vi "Mindsensors SumoEyes Config.vi"(10 "Node Data":T2) -> ()   [LabVIEW 2010]
uses:
  Datatypes/Node.ctl
  UI Controls/PlugInControls/Pluginbackground.ctl
  <vilib>/NXT/Subs/LVHSConnector.ctl
  <vilib>/Utility/miscctls.llb/LVPointTypeDef.ctl
  <vilib>/NXT/Block Support/HWPage.SensorMode.ctl
  <vilib>/NXT/Block Support/HWPage.SensorType.ctl
  ConvertNodeAddrSensor.vi
  SavePendingGlobal.vi
panel:
  in  "Ring":u16(ring)=5 items=["short"=5, "long"=6]
  out "?":ext format="%#.2g"
  in  "NXT Port":string
  out "Both 2":bool
  out "Right 2":bool
  out "Left 2":bool
  out "Both":bool
  out "Right":bool
  out "Left":bool
  in  "Range":string
  out "Reading":i16=45
  in  "NXT":T1
  in  "Name":string
  out "Headline":string="Type (auto populated)"
  in  "Sensor Parameters":string
  in  "Reset":bool
  in  "Save":bool
  in  "Stop":bool
  out "Background":T3=TRUE
  # "<- No controls below this line"
  # "Common controls such as Buttons, Rings, Sliders, Graphs, Decorations, etc can be found in the <labview>\\Targets\\NI\\NXT\\NXT Toolkit\\Schematic Editor\\UI Controls\\Plugin Controls\\ folder. Use these controls when possible to ensure a consistent look and feel with LabVIEW Education Edition."
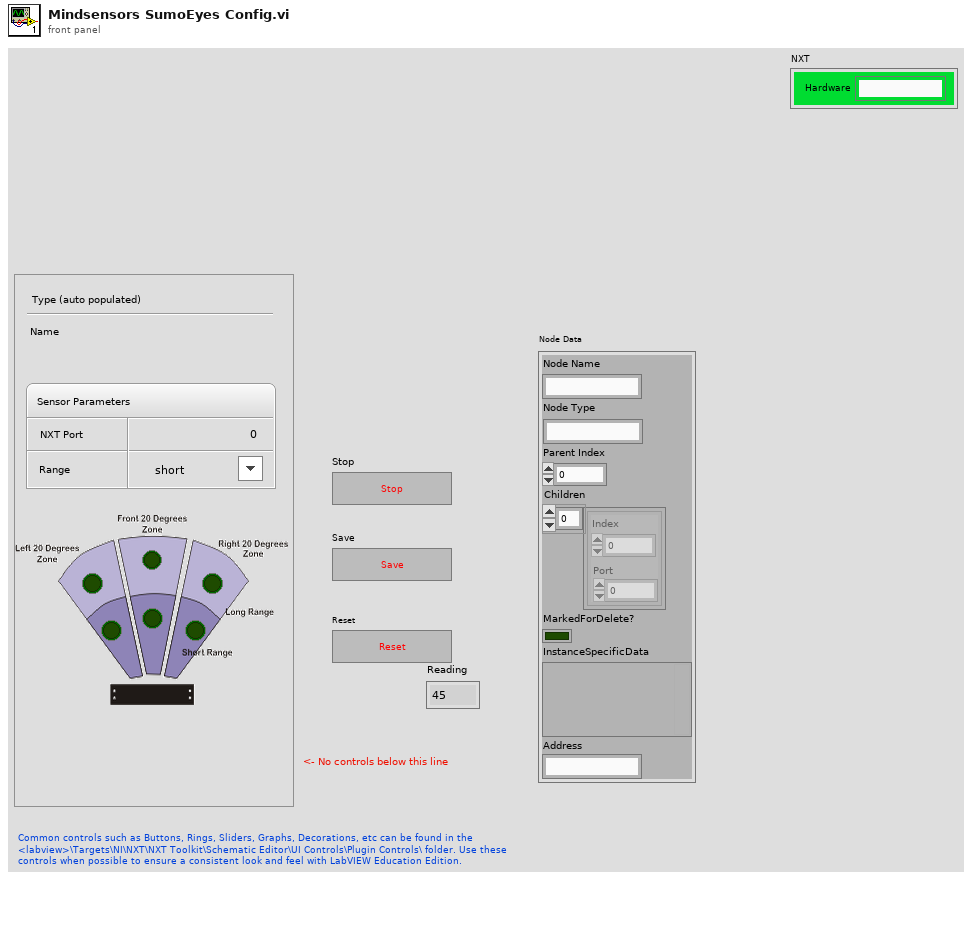
[diagram p1: front panel]
types:
  T1 = typedef "LVHSConnector.ctl" = cluster{"Hardware":string, "Flattened String":string}
  T2 = typedef "Node.ctl" = cluster{"Node Name":string, "Node Type":string, "Parent Index":i16, "Children":cluster{"Index":u16, "Port":u16}[], "MarkedForDelete?":bool, "InstanceSpecificData":variant, "Address":string}
  T3 = typedef "Pluginbackground.ctl" = bool
  T4 = typedef "LVPointTypeDef.ctl" = cluster{"Horizontal":i16, "Vertical":i16}
  T5 = enum8{"Enabled", "Disabled", "Disabled and Grayed Out"}
  T6 = typedef "HWPage.SensorMode.ctl" = u8
  T7 = typedef "HWPage.SensorType.ctl" = u8
  T8 = typedef "NXT_InputPort.ctl" = u8
  T9 = typedef "nxt.ctl" = cluster{"nxtHandle":u32, "fileHandle":u32, "fileIterHandle":u32, "moduleHandle":u32, "modIterHandle":u32, "nxtIterHandle":u32}
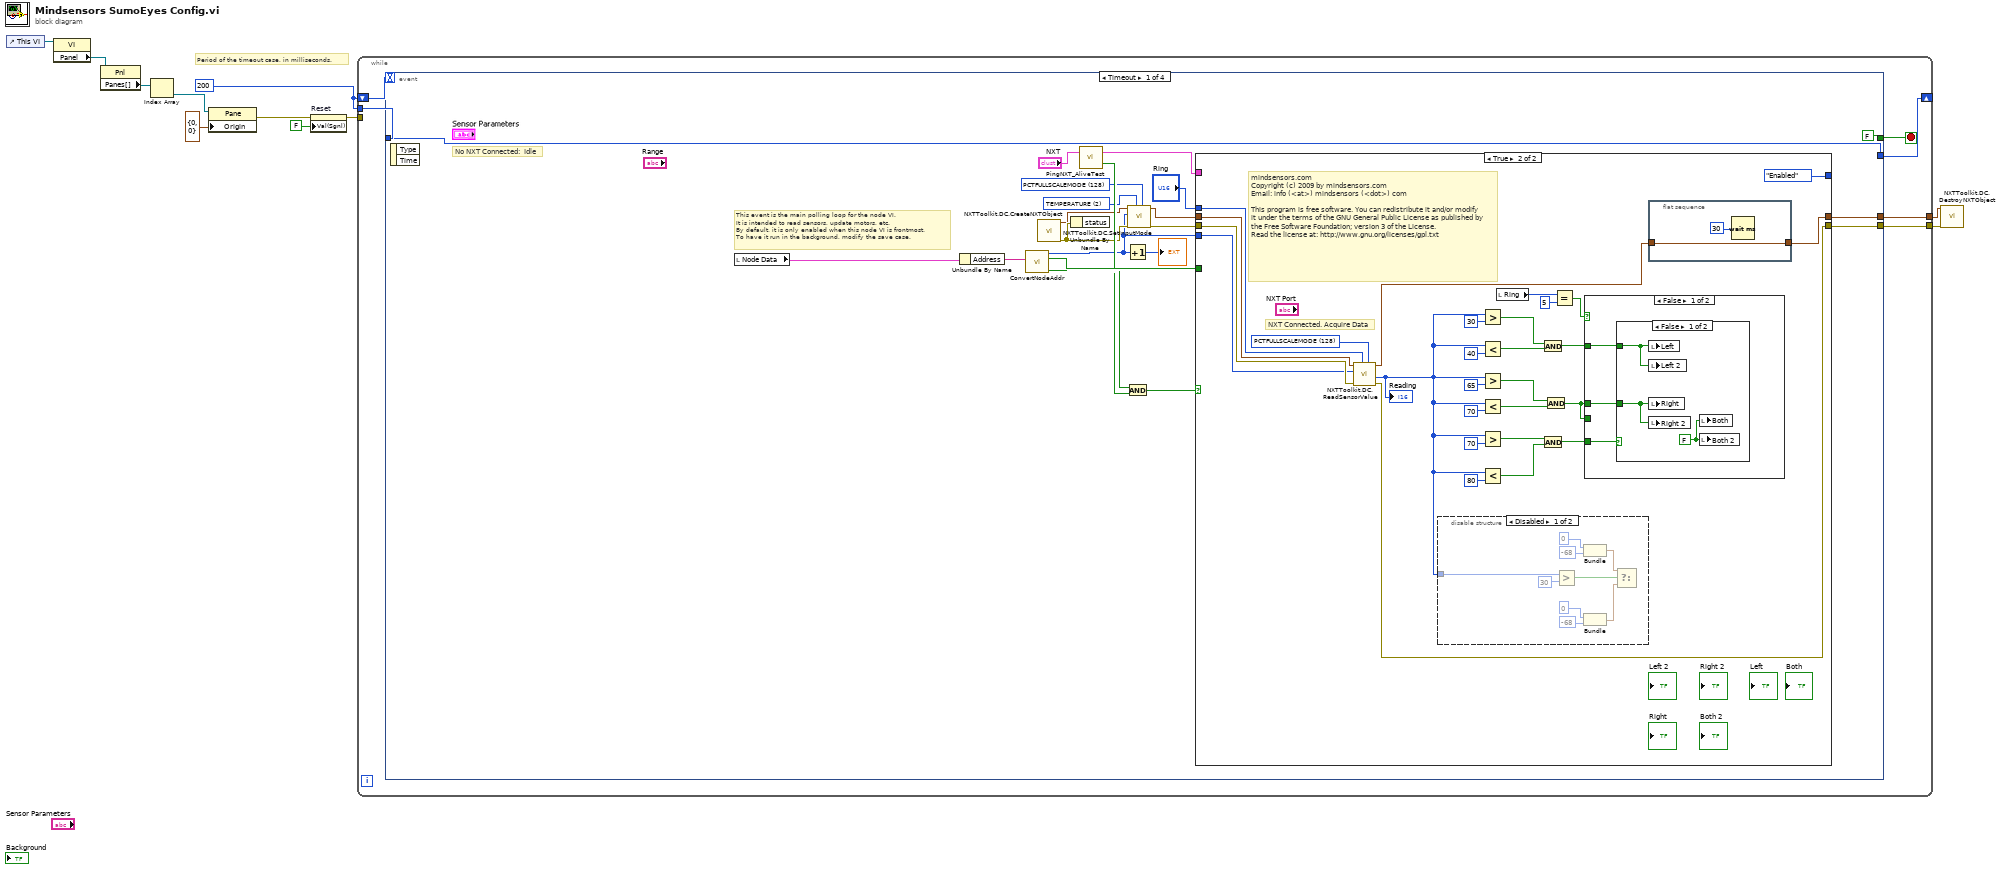
[diagram p0: block diagram]
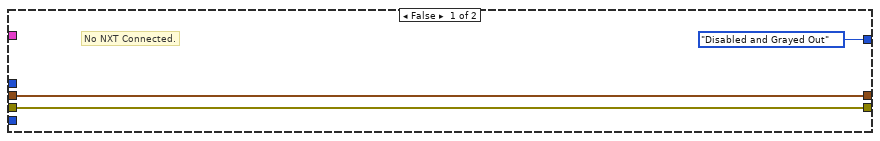
[diagram p2: hidden frame]
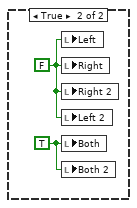
[diagram p3: hidden frame]
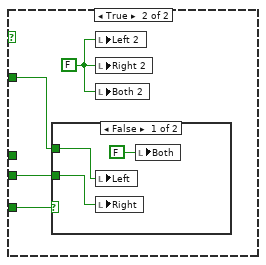
[diagram p4: hidden frame]
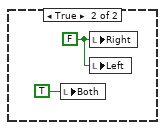
[diagram p5: hidden frame]
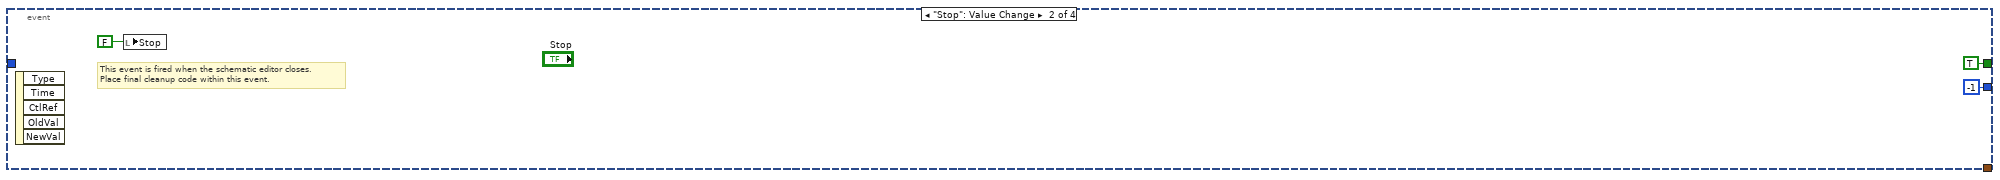
[diagram p7: hidden frame]
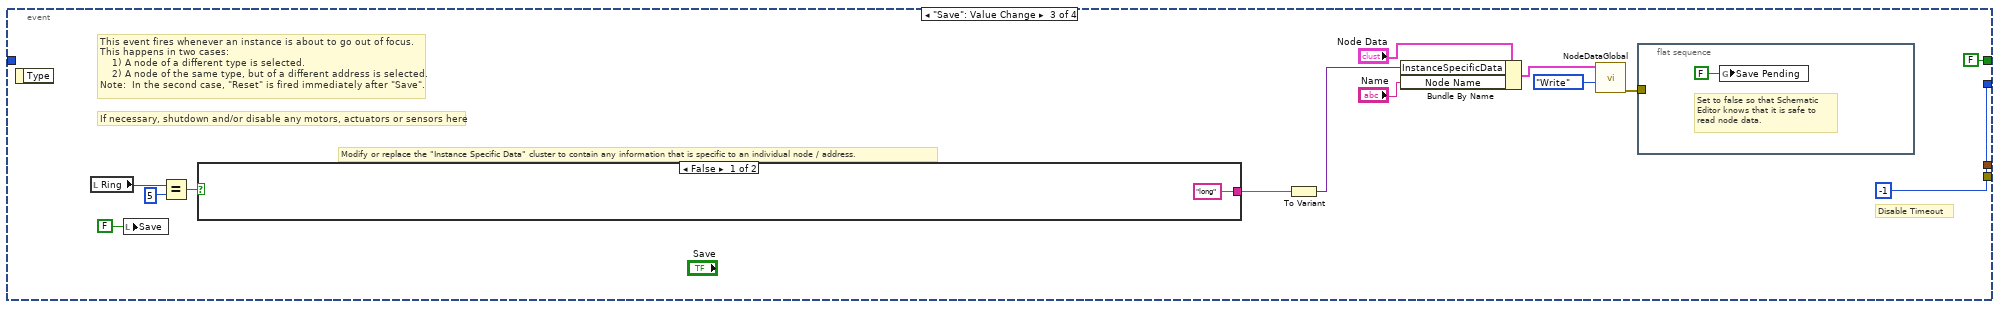
[diagram p8: hidden frame]
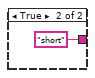
[diagram p9: hidden frame]
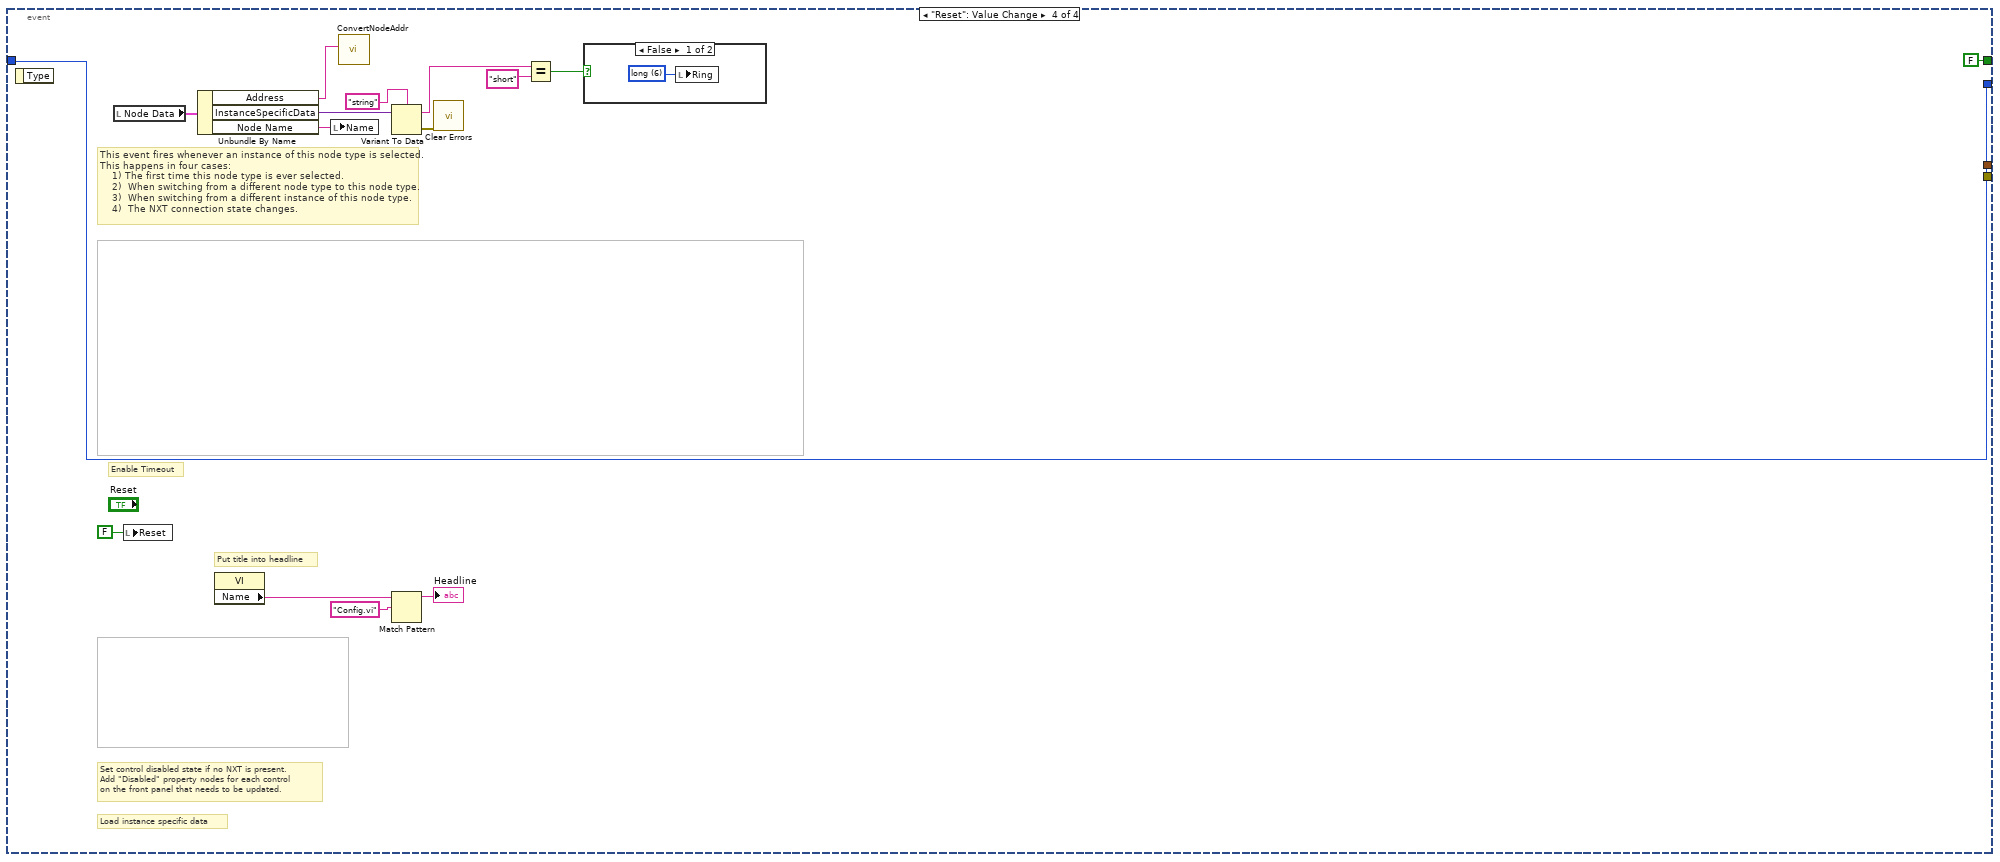
[diagram p10: hidden frame]
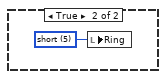
[diagram p11: hidden frame]
diagram:
  w10 = 200
  # "Period of the timeout case, in milliseconds."
  n1 = control-ref of="This VI"() -> (w5:refnum<vi>)
  n2 = property class="VI"(reference=w5) -> ("Panel"=w6:refnum<vi>)  [unwired: 1 in, 2 out]
  n3 = property class="Pnl"(reference=w6) -> ("Panes[]"=w7:refnum<vi>[])  [unwired: 1 in, 2 out]
  n4 = Index Array(array=w7) -> (element=w8:refnum<vi>)  [unwired: 1 in]
  n5 = property class="Pane"(reference=w8, "Origin"=T4 {"Horizontal"=0, "Vertical"=0}) -> (error out=w4:errorcluster)  [unwired: 1 in, 1 out]
  n6 = property on="Reset" class="Bool (strict)"(error in=w4, "Val(Sgnl)"=FALSE ("Value (Signaling)")) -> (error out=w11:errorcluster)  [unwired: 1 in, 1 out]
  n7 = while {
    tunnel: w11 -> [_]
    shift-right: [w15] -> _
    shift-left: w10 -> [w16]
    tunnel: w10 -> [w14]
    tunnel: [w13] -> w2
    tunnel: [w12] -> w1
    stop <- w17 stop-if-true
    n8 = event shown="[0] Timeout" {
      selector: _ -> [_ _ _ _]
      dyn-events: _ -> [_ _ _ _]
      timeout: w16 -> [_ _ _ _]
      tunnel: [FALSE TRUE FALSE FALSE] -> w17
      tunnel: [w37 -1 -1 w127] -> w15
      tunnel: w14 -> [w37 _ _ w127]
      tunnel: [w23 _ _ _] -> w13
      tunnel: [w22 _ _ _] -> w12
      event Timeout {
        w26 = T6 128 items=["RAWMODE"=0, "BOOLEANMODE"=32, "TRANSITIONCNTMODE"=64, "PERIODCOUNTERMODE"=96, "PCTFULLSCALEMODE"=128, "CELSIUSMODE"=160, "FAHRENHEITMODE"=192, "ANGLESTEPMODE"=224] ("Sensor Mode (RAWMODE)")
        w27 = T7 2 items=["NO_SENSOR", "SWITCH", "TEMPERATURE", "REFLECTION", "ANGLE", "LIGHT_ACTIVE", "LIGHT_INACTIVE", "SOUND_DB", "SOUND_DBA", "CUSTOM", "LOWSPEED", "LOWSPEED_9V", "HIGHSPEED"] ("Sensor Type (NO_SENSOR)")
        # "No NXT Connected:  Idle"
        # "This event is the main polling loop for the node VI.\nIt is intended to read sensors, update motors, etc.\nBy default, it is only enabled when this node VI is frontmost.\nTo have it run in the background, modify the save case."
        n9 = event-data() -> ()  [unwired: 1 in, 2 out]
        n10 = local read "Node Data"() -> (w30:T2)
        n11 = Unbundle By Name(w30) -> ("Address"=w34:string)
        n12 = call-poly "ConvertNodeAddr.vi"("Sensor Port"=w34) -> ("Valid Addr?"=w35:bool, "MUX Present?"=w36:bool, "NXT Port"=w18:T8)  [unwired: 6 in, 2 out]
        n13 = call <vilib>:"NXTToolkit.DC.CreateNXTObject.vi"() -> ("error out"=w29:errorcluster, "NXTObject"=w28:T9)  [unwired: 9 in, 1 out]
        n14 = Unbundle By Name(w29) -> ()  [unwired: 1 out]
        n15 = call <vilib>:"PingNXT_AliveTest.vi"("NXT"="NXT") -> ("connected?"=w33:bool, "NXT"=w32:T1)  [unwired: 1 in]
        n16 = Increment(x=w18) -> (x+1=→"?":T8)
        n17 = And(x=w35, y=w33) -> (x .and. y?=w21:bool)
        n18 = call <vilib>:"NXTToolkit.DC.SetInputMode.vi"("Sensor Mode (RAWMODE)"=w26, "Sensor Type (NO_SENSOR)"=w27, "error in (no error)"=w29, "Input Port (Port 1)"=w18, "NXTObject"=w28) -> ("error out"=w24:errorcluster, "NXTObject dup"=w25:T9)  [unwired: 4 in, 1 out]
        n19 = case shown="True" w21 {
          tunnel: w32 -> [_ _]
          tunnel: w36 -> [_ _]
          tunnel: [T5."Disabled and Grayed Out" ("Disabled") T5."Enabled" ("Disabled")] -> _
          tunnel: w25 -> [w40 w69]
          tunnel: w24 -> [w39 w68]
          tunnel: [w40 w51] -> w23
          tunnel: [w39 w50] -> w22
          tunnel: w18 -> [_ w49]
          tunnel: "Ring" -> [_ w48]
          frame False {
            # "No NXT Connected."
          }
          frame True {
            w66 = T6 128 items=["RAWMODE"=0, "BOOLEANMODE"=32, "TRANSITIONCNTMODE"=64, "PERIODCOUNTERMODE"=96, "PCTFULLSCALEMODE"=128, "CELSIUSMODE"=160, "FAHRENHEITMODE"=192, "ANGLESTEPMODE"=224] ("Sensor Mode (RAWMODE)")
            # "mindsensors.com\nCopyright (c) 2009 by mindsensors.com\nEmail: info (<at>) mindsensors (<dot>) com\n\nThis program is free software. You can redistribute it and/or modify\nit under the terms of the GNU General Public License as published by\nthe Free Software Foundation; version 3 of the License.\nRead the license at: http://www.gnu.org/licenses/gpl.txt"
            # "NXT Connected. Acquire Data"
            n20 = call <vilib>:"NXTToolkit.DC.ReadSensorValue.vi"("Sensor Mode (RAWMODE)"=w66, "SensorType (NO_SENSOR)"=w48, "error in (no error)"=w68, "Input Port (Port 1)"=w49, "NXTObject"=w69) -> ("error out"=w50:errorcluster, "Scaled Value"=w53:i16, "NXTObject dup"=w67:T9)  [unwired: 1 in, 3 out]
            "Reading" <- w53
            n21 = disable-structure shown="Disabled" {
              disable-tunnel: w53 -> [w87 _]
              frame Disabled {
                n22 = Greater?(x=w87, y=i16 30) -> (0:w88:bool)
                n23 = Bundle(0, -68) -> (w92:cluster{i32, i32})  [unwired: 1 in]
                n24 = Bundle(0, -68) -> (w89:cluster{i32, i32})  [unwired: 1 in]
                n25 = Select(t=w92, s=w88, f=w89) -> ()  [unwired: 1 out]
              }
              frame Enabled {
              }
            }
            n26 = Greater?(x=w53, y=u8 30 ("x")) -> (0:w55:bool)
            n27 = Less?(x=w53, y=u8 40) -> (x < y?=w54:bool)
            n28 = Greater?(x=w53, y=u8 65 ("x")) -> (0:w59:bool)
            n29 = Less?(x=w53, y=u8 70) -> (x < y?=w58:bool)
            n30 = Greater?(x=w53, y=u8 70 ("x")) -> (0:w63:bool)
            n31 = Less?(x=w53, y=u8 80) -> (x < y?=w62:bool)
            n32 = local read "Ring"() -> (w46:u16)
            n33 = And(x=w55, y=w54) -> (x .and. y?=w52:bool)
            n34 = And(x=w63, y=w62) -> (x .and. y?=w43:bool)
            n35 = And(x=w59, y=w58) -> (x .and. y?=w42:bool)
            n36 = Equal?(x=w46, y=u16 5) -> (x = y?=w44:bool)
            n37 = case shown="False" w44 {
              tunnel: w52 -> [w72 w81]
              tunnel: w42 -> [_ w80]
              tunnel: w43 -> [w71 w79]
              tunnel: w42 -> [w70 _]
              frame False {
                n38 = case shown="False" w71 {
                  tunnel: w72 -> [w74 _]
                  tunnel: w70 -> [w73 _]
                  frame False {
                    w75 = FALSE ("Boolean 4")
                    n39 = local write "Left"(w74) -> ()
                    n40 = local write "Left 2"(w74) -> ()
                    n41 = local write "Right"(w73) -> ()
                    n42 = local write "Right 2"(w73) -> ()
                    n43 = local write "Both"(w75) -> ()
                    n44 = local write "Both 2"(w75) -> ()
                  }
                  frame True {
                    w77 = FALSE
                    w76 = TRUE
                    n45 = local write "Left"(w77) -> ()
                    n46 = local write "Right"(w77) -> ()
                    n47 = local write "Right 2"(w77) -> ()
                    n48 = local write "Left 2"(w77) -> ()
                    n49 = local write "Both"(w76) -> ()
                    n50 = local write "Both 2"(w76) -> ()
                  }
                }
              }
              frame True {
                w78 = FALSE ("Both 2")
                n51 = case shown="False" w79 {
                  tunnel: w81 -> [w82 _]
                  tunnel: w80 -> [w83 _]
                  frame False {
                    n52 = local write "Left"(w82) -> ()
                    n53 = local write "Right"(w83) -> ()
                    n54 = local write "Both"(FALSE ("Boolean 4")) -> ()
                  }
                  frame True {
                    w85 = FALSE
                    n55 = local write "Both"(TRUE) -> ()
                    n56 = local write "Right"(w85) -> ()
                    n57 = local write "Left"(w85) -> ()
                  }
                }
                n58 = local write "Left 2"(w78) -> ()
                n59 = local write "Right 2"(w78) -> ()
                n60 = local write "Both 2"(w78) -> ()
              }
            }
            n61 = flat-sequence {
              tunnel: [w96] -> w51
              tunnel: w67 -> [w96]
              frame #0 {
                n62 = Wait (ms)(milliseconds to wait=u32 30) -> ()  [unwired: 1 out]
              }
            }
          }
        }
      }
      event "Stop": Value Change {
        # "This event is fired when the schematic editor closes.\nPlace final cleanup code within this event."
        n63 = event-data() -> ()  [unwired: 1 in, 5 out]
        n64 = local write "Stop"(FALSE ("stop")) -> ()
      }
      event "Save": Value Change {
        # "If necessary, shutdown and/or disable any motors, actuators or sensors here"
        # "Modify or replace the \"Instance Specific Data\" cluster to contain any information that is specific to an individual node / address."
        # "Disable Timeout"
        # "This event fires whenever an instance is about to go out of focus.\nThis happens in two cases:\n    1) A node of a different type is selected.\n    2) A node of the same type, but of a different address is selected.\nNote:  In the second case, \"Reset\" is fired immediately after \"Save\"."
        n65 = event-data() -> ()  [unwired: 1 in, 1 out]
        n66 = local read "Ring"() -> (w104:u16)
        n67 = local write "Save"(FALSE ("stop")) -> ()
        n68 = Equal?(x=w104, y=u16 5) -> (x = y?=w101:bool)
        n69 = case shown="False" w101 {
          tunnel: ["long" ("Name 2") "short" ("Name 2")] -> w102
          frame False {
          }
          frame True {
          }
        }
        n70 = To Variant(anything=w102) -> (Variant=w111:variant)
        n71 = Bundle By Name(cluster="Node Data", "InstanceSpecificData"=w111, "Node Name"="Name") -> (w110:T2)
        n72 = call "NodeDataGlobal.vi"("Action"=enum16{"Read", "Write"}."Write", "Node Data In"=w110) -> ("error out"=w105:errorcluster)  [unwired: 8 in, 1 out]
        n73 = flat-sequence {
          tunnel: w105 -> [_]
          frame #0 {
            # "Set to false so that Schematic\nEditor knows that it is safe to\nread node data."
            n74 = global write "SavePendingGlobal.vi" "Save Pending"(FALSE ("Save Pending")) -> ()
          }
        }
      }
      event "Reset": Value Change {
        # "Set control disabled state if no NXT is present.\nAdd \"Disabled\" property nodes for each control\non the front panel that needs to be updated."
        # "Load instance specific data"
        # "Enable Timeout"
        # "This event fires whenever an instance of this node type is selected.\nThis happens in four cases:\n    1) The first time this node type is ever selected.\n    2)  When switching from a different node type to this node type.\n    3)  When switching from a different instance of this node type. \n    4)  The NXT connection state changes."
        # "Put title into headline"
        n75 = event-data() -> ()  [unwired: 1 in, 1 out]
        n76 = local read "Node Data"() -> (w128:T2)
        n77 = local write "Reset"(FALSE ("Reset")) -> ()
        n78 = Unbundle By Name(w128) -> ("Address"=w121:string, "InstanceSpecificData"=w129:variant, "Node Name"=w122:string)
        n79 = property class="VI"() -> ("Name"=w124:string)  [unwired: 2 in, 2 out]
        n80 = local write "Name"(w122) -> ()
        n81 = call-poly "ConvertNodeAddr.vi"("Sensor Port"=w121) -> ()  [unwired: 6 in, 5 out]
        n82 = Variant To Data(Variant=w129, type="string") -> (error out=w126:errorcluster, data=w119:string)  [unwired: 1 in]
        n83 = Match Pattern(string=w124, regular expression="Config.vi") -> (before substring=→"Headline":string)  [unwired: 1 in, 3 out]
        n84 = call <vilib>:"Clear Errors.vi"("error in (no error)"=w126) -> ()  [unwired: 6 in, 1 out]
        n85 = Equal?(x=w119, y="short") -> (x = y?=w117:bool)
        n86 = case shown="False" w117 {
          frame False {
            w132 = u16 6 items=["short"=5, "long"=6] ("Ring")
            n87 = local write "Ring"(w132) -> ()
          }
          frame True {
            w133 = u16 5 items=["short"=5, "long"=6] ("Ring")
            n88 = local write "Ring"(w133) -> ()
          }
        }
      }
    }
  }
  n89 = call <vilib>:"NXTToolkit.DC.DestroyNXTObject.vi"("error in (no error)"=w1, "NXTObject"=w2) -> ()  [unwired: 9 in, 1 out]
